vi "HK Item Check Alarm.vi"(8 "error in (no error)":errorcluster, 10 "Value":dbl, 11 "HK Item in":refnum<class "HK Item.lvclass">) -> (0 "error out":errorcluster, 2 "Alarm Status":T1, 3 "HK Item out":refnum<class "HK Item.lvclass">)   [LabVIEW 2024, in "HK Item.lvclass"]
uses:
  HK Item.lvclass
  HK Alarms/HK Alarm enum Status.ctl
  HK Item.lvclass/HK Item.ctl
  HK Alarms/HK Alarms.lvclass
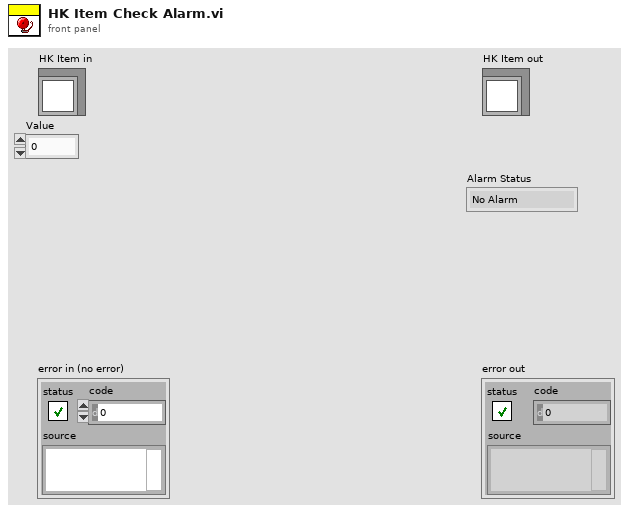
[diagram p1: front panel]
types:
  T1 = typedef "HK Item.lvclass/HK Alarm enum Status.ctl" = enum16{"No Alarm", "Red Low", "Red High", "Yellow Low", "Yellow High"}
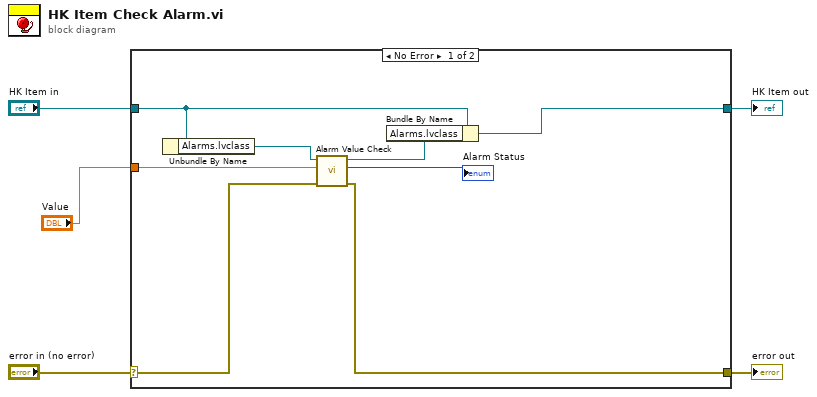
[diagram p0: block diagram]
diagram:
  n1 = case shown="No Error" "error in (no error)" {
    selector: "error in (no error)" -> [w11 w15]
    tunnel: [w10 w15] -> w4
    tunnel: [w7 w14] -> w2
    tunnel: "HK Item in" -> [w6 w14]
    tunnel: "Value" -> [w12 _]
    frame No Error {
      n2 = Unbundle By Name(w6) -> ("Alarms.lvclass"=w13:refnum<class "HK Alarms.lvclass">)
      n3 = call-dynamic "Alarm Value Check.vi"("error in (no error)"=w11, "Value"=w12, "HK Alarms in"=w13) -> ("error out"=w10:errorcluster, "Alarm Status"=→"Alarm Status":T1, "HK Alarms out"=w9:refnum<class "HK Alarms.lvclass">)  [unwired: 6 in]
      n4 = Bundle By Name(cluster=w6, "Alarms.lvclass"=w9) -> (w7:refnum<class "HK Item.lvclass">)
    }
    frame Error {
    }
  }
  "error out" <- w4
  "HK Item out" <- w2
